vi "quat2eulerXYZ.vi"(11 "Quaternions":dbl[](array[numeric])) -> (3 "Euler Angles [rad]":cluster{"phi":dbl, "theta":dbl, "psi":dbl})   [LabVIEW 2017]
uses:
  <vilib>/Analysis/coordinate.llb/Euler Rotation Order.ctl
  <vilib>/Analysis/NI_AALPro.lvlib
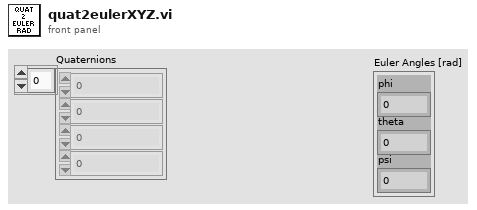
[diagram p1: front panel]
types:
  T1 = typedef "NI_AALPro.lvlib/Euler Rotation Order.ctl" = u16
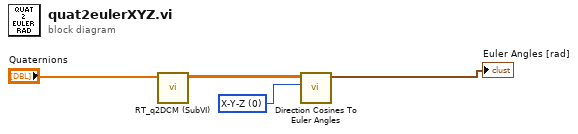
[diagram p0: block diagram]
diagram:
  w2 = T1 0 items=["X-Y-Z", "X-Z-Y", "Y-X-Z", "Y-Z-X", "Z-X-Y", "Z-Y-X", "X-Y-X", "X-Z-X", "Y-X-Y", "Y-Z-Y", "Z-X-Z", "Z-Y-Z"] ("rotation order")
  n1 = call "RT_q2DCM (SubVI).vi"("Quaternion"="Quaternions") -> ("DCM"=w3:dbl[][])  [unwired: 10 in]
  n2 = call <vilib>:"Direction Cosines To Euler Angles.vi"("rotation order"=w2, "Direction Cosines"=w3) -> ("Euler Angles"=→"Euler Angles [rad]":cluster{"phi":dbl, "theta":dbl, "psi":dbl})  [unwired: 8 in, 1 out]
